vi "Send Set Ratios.vi"(7 "Message Priority (Normal)":T1=enum."Normal", 8 "error in (no error)":errorcluster, 9 "Start Index":i32, 10 "PWM Ratios":dbl[](array[numeric]) format="%.3g", 11 "Message Enqueuer":refnum<class "Message Enqueuer.lvclass">) -> (0 "error out":errorcluster, 3 "Message Enqueuer out":refnum<class "Message Enqueuer.lvclass">)   [LabVIEW 2020, in "BNT_ULx.lvlib" / "Set Ratios Msg.lvclass"]
doc: "Sends the <B>BNT_ULx.lvlib:Set Ratios Msg.lvclass</B> message.\n\n<B>BNT_DAQmx.lvlib:BNT_DAQmx-MCSV-DOPWM.lvclass:Set Ratios.vi</B> Description:\n\nSet pulse width ratios."
uses:
  Set Ratios Msg.lvclass
  <vilib>/ActorFramework/Message Enqueuer/Message Enqueuer.lvclass
  <vilib>/ActorFramework/Message Enqueuer/Message Priority.ctl
  C:/Program Files (x86)/National Instruments/LabVIEW 2020/vi.lib/ActorFramework/Message/Message.lvclass
  Set Ratios Msg.lvclass/Set Ratios Msg.ctl
  <vilib>/ActorFramework/Message Enqueuer/Message Enqueuer.lvclass/Message Enqueuer.ctl
  <vilib>/ActorFramework/Message Priority Queue/Priority Enqueue.vi
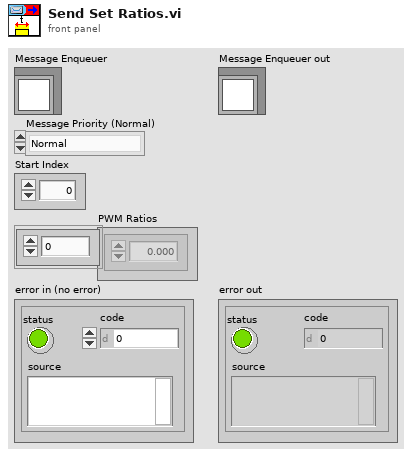
[diagram p1: front panel]
types:
  T1 = typedef "Actor Framework.lvlib/Message Enqueuer.lvclass/Message Priority.ctl" = enum16{"Low", "Normal", "High"}
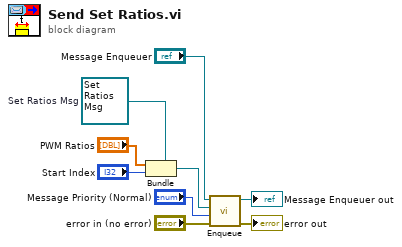
[diagram p0: block diagram]
diagram:
  w3 = refnum<class "Set Ratios Msg.lvclass"> refnum  # Set Ratios Msg
  n1 = Bundle(cluster=w3, "PWM Ratios", "Start Index") -> (w6:refnum<class "Set Ratios Msg.lvclass">)
  n2 = call <vilib>:"Enqueue.vi"("error in (no error)"="error in (no error)", "Message Priority (Normal)"="Message Priority (Normal)", "Message"=w6, "Message Enqueuer in"="Message Enqueuer") -> ("error out"=→"error out":errorcluster, "Message Enqueuer out"=→"Message Enqueuer out":refnum<class "Message Enqueuer.lvclass">)  [unwired: 6 in]
